vi "Read item.vi"(0 "data in":string) -> (3 "Test Item name":string[](array[string]), 4 "after substring":string, 5 "Seq numbers":i32, 6 "输出数组":string[][](array[string]))   [LabVIEW 2018]
panel:
  out "data in 2":string
  out "Nxt.Name":string[](array[string])
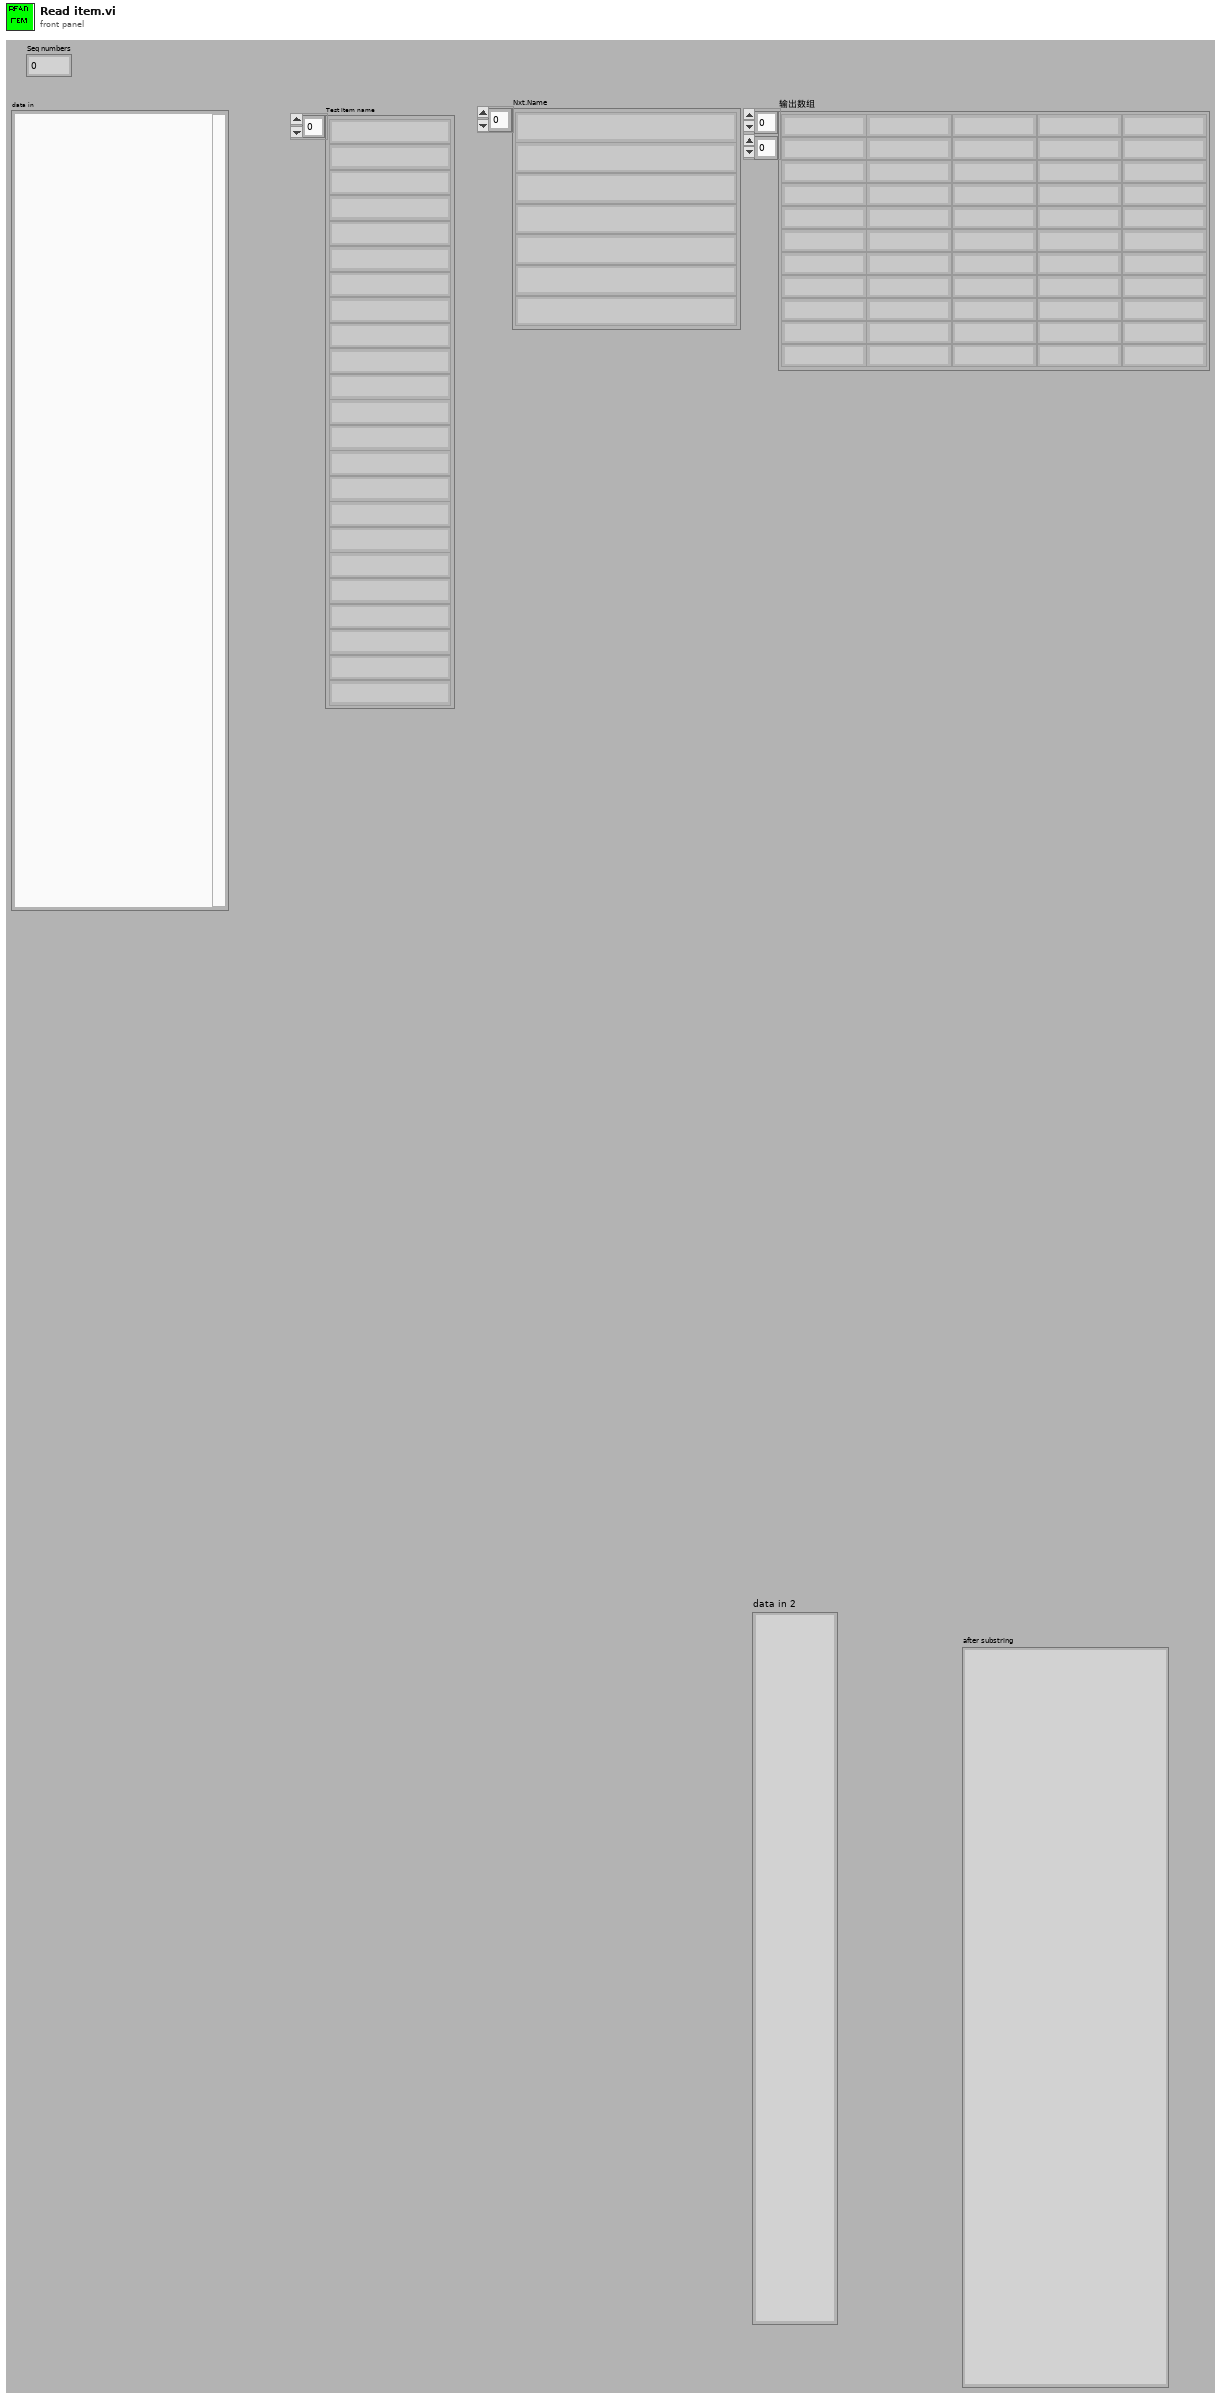
[diagram p1: front panel]
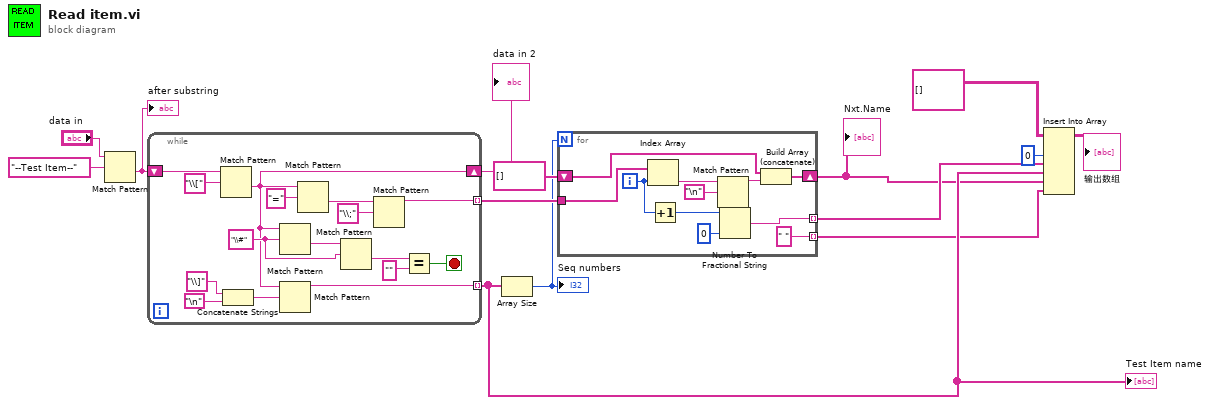
[diagram p0: block diagram]
diagram:
  n1 = Match Pattern(string="data in", regular expression="--Test Item--") -> (after substring=w13:string)  [unwired: 4 out]
  "after substring" <- w13
  n2 = while {
    shift-right: [w25] -> w8
    shift-left: w13 -> [w15]
    tunnel: [w23] -> w3 mode=indexing
    tunnel: [w20] -> w11 mode=indexing
    stop <- w17 stop-if-true
    w26 = "\\#" ("regular expression")
    n3 = Match Pattern(string=w15, regular expression="\\[") -> (after substring=w25:string)  [unwired: 4 out]
    n4 = Concatenate Strings("\\]", "\n") -> (w16:string)
    n5 = Match Pattern(string=w25, regular expression=w26) -> (after substring=w27:string)  [unwired: 4 out]
    n6 = Match Pattern(string=w25, regular expression=w16) -> (before substring=w23:string)  [unwired: 4 out]
    n7 = Match Pattern(string=w25, regular expression="=") -> (after substring=w22:string)  [unwired: 4 out]
    n8 = Match Pattern(string=w27, regular expression=w26) -> (after substring=w19:string)  [unwired: 4 out]
    n9 = Match Pattern(string=w22, regular expression="\\;") -> (before substring=w20:string)  [unwired: 4 out]
    n10 = Equal?(x=w19, y="") -> (x = y?=w17:bool)
  }
  "Test Item name" <- w3
  "data in 2" <- w8
  n11 = Array Size(array=w3) -> (size(s)=w9:i32)
  "Seq numbers" <- w9
  n12 = for {
    N: w9 -> [_]
    tunnel: w11 -> [w40]
    shift-right: [w37] -> w2
    shift-left: string[] [] -> [w36]
    tunnel: [w33] -> w4 mode=indexing
    tunnel: [" "] -> w1 mode=indexing
    i -> [w35]
    n13 = Index Array(array=w40, index=w35) -> (element=w39:string)
    n14 = Increment(x=w35) -> (x+1=w32:i32)
    n15 = Match Pattern(string=w39, regular expression="\n") -> (before substring=w38:string)  [unwired: 4 out]
    n16 = Number To Fractional String(number=w32, precision (6)=i16 0 ("精度(6)")) -> (F-format string=w33:string)  [unwired: 2 in]
    n17 = Build Array (concatenate)(w36, w38) -> (w37:string[])
  }
  "Nxt.Name" <- w2
  n18 = Insert Into Array(array=string[][] [], index (col)=0 ("禁用的索引 (列)"), new element #1=w4, new element #2=w3, new element #3=w2, new element #4=w1) -> (→"输出数组":string[][])  [unwired: 1 in]
